vi "GetQueue.vi"(7 "Instance":i32, 8 "error in (no error)":errorcluster) -> (0 "error out":errorcluster, 1 "Event?":bool, 2 "queue out":refnum<queue>)   [LabVIEW 2017, in "Communication.lvlib"]
uses:
  Communication.lvlib
  MsgData.ctl
  MsgAck.ctl
  QueueRepo.Action.ctl
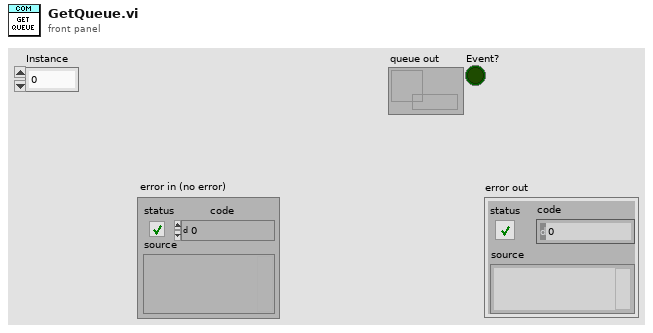
[diagram p1: front panel]
types:
  T1 = typedef "Communication.lvlib/QueueRepo.Action.ctl" = enum16{"Add", "Get", "Destroy", "Get All", "Clear"}
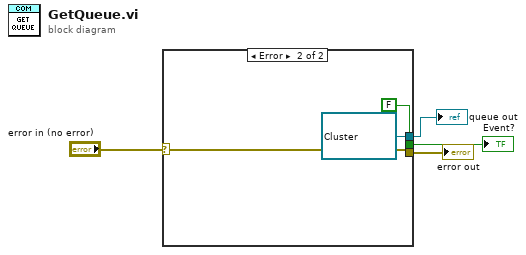
[diagram p0: block diagram]
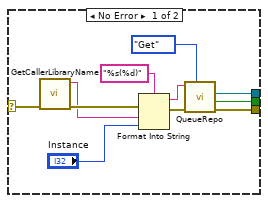
[diagram p2: hidden frame]
diagram:
  n1 = case shown="Error" "error in (no error)" {
    selector: "error in (no error)" -> [w15 w18]
    tunnel: [w9 w18] -> w3
    tunnel: [w6 refnum<queue> refnum ("queue out")] -> w2
    tunnel: [w5 FALSE ("Event?")] -> w1
    frame No Error {
      n2 = call "GetCallerLibraryName.vi"("error in (no error)"=w15) -> ("error out"=w14:errorcluster, "Name"=w13:string)  [unwired: 9 in]
      n3 = Format Into String(format string="%s(%d)", error in=w14, w13, "Instance") -> (resulting string=w8:string, error out=w10:errorcluster)  [unwired: 1 in]
      n4 = call "QueueRepo.vi"("Action"=QueueRepo.Action."Get", "error in (no error)"=w10, "Name"=w8) -> ("error out"=w9:errorcluster, "Event?"=w5:bool, "queue out"=w6:refnum<queue>)  [unwired: 5 in, 1 out]
    }
    frame Error {
    }
  }
  "error out" <- w3
  "queue out" <- w2
  "Event?" <- w1
